vi "Check ref frame has been selected.vi"(6 "Case name string":string, 8 "error in (no error)":errorcluster) -> (0 "error out":errorcluster, 3 "Proceed / Reference frame has been selected":bool)   [LabVIEW 2017]
uses:
  Typedefs/Top level VI states.ctl
  Global Variables/General Globals.vi
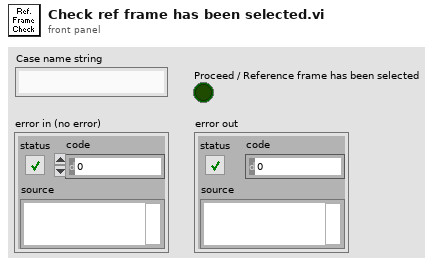
[diagram p1: front panel]
types:
  T1 = typedef "Top level VI states.ctl" = enum16{"None", "Initialise UI", "<STACK PROTOCOL STATES>", "AOL Zstack-START", "AOL Zstack-STOP", "Motor Zstack-START", "Motor Zstack-STOP", "Parameter Sweep-START", "Parameter Sweep-STOP", "<ACQUISITION PROTOCOL STATES> ", "Functional Acquisition-START", "Functional Acquisition-STOP", "Single Plane Acquisition-START", "Single Plane Acquisition-STOP", "Volume Acquisition-START", "Volume Acquisition-STOP", "<LIVE IMAGING PROTOCOL STATES>", "Live Imaging-START", "Live Imaging-STOP", "Live Plane Imaging-START", "Live Plane Imaging-STOP", "Live Volume Imaging-START", "Live Volume Imaging-STOP", "<MOVEMENT CORRECTION PROTOCOL STATES>", "EXIT"}
  T2 = typedef "Reference_Globals.ctl" = cluster{"Refrence data path":path, "Reference Rectangle":i16[][], "AOL Z":dbl, "No of pixels in a miniscan ":i32[], "Threshold":i16[], "No of miniscans":i32[], "Full Frame Size":u16, "Reference Image":T3, "dwelltime":dbl, "Zoom":dbl, "Field of View":dbl, "Z Step":i8, "Z pixels":i32, "Z Lines":u8, "Z Ignore":u8, "Laser":u8}
  T3 = typedef "IMAQ Image.ctl" = refnum<image>
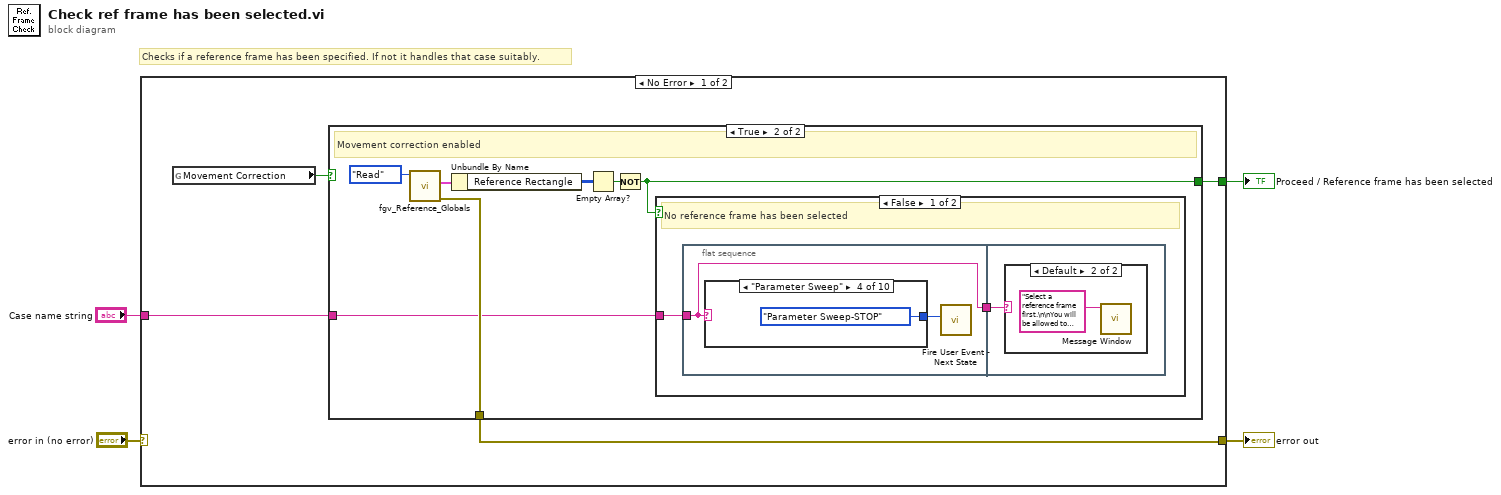
[diagram p0: block diagram]
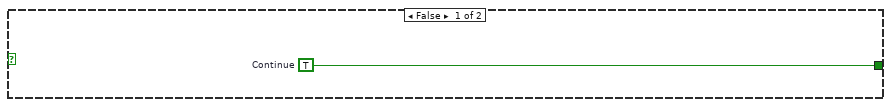
[diagram p2: hidden frame]
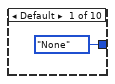
[diagram p3: hidden frame]
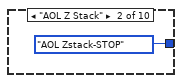
[diagram p4: hidden frame]
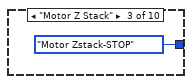
[diagram p5: hidden frame]
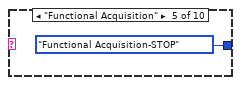
[diagram p6: hidden frame]
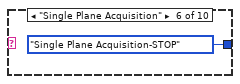
[diagram p7: hidden frame]
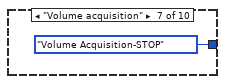
[diagram p8: hidden frame]
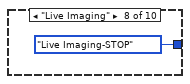
[diagram p9: hidden frame]
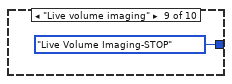
[diagram p10: hidden frame]
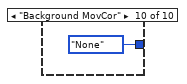
[diagram p11: hidden frame]
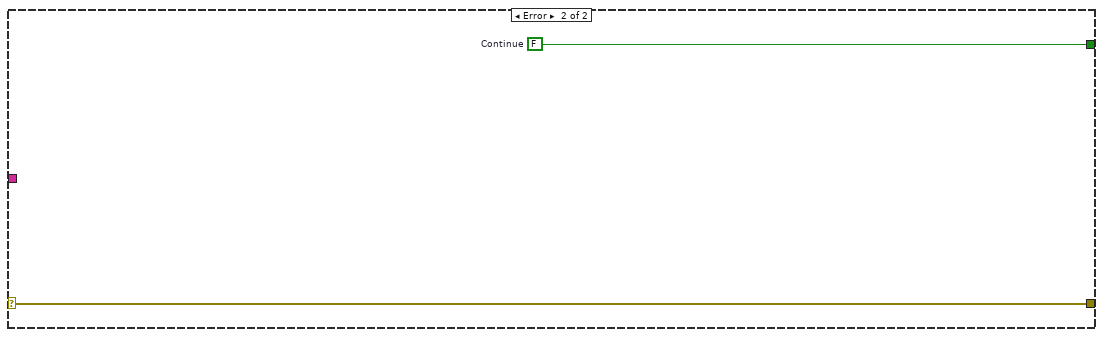
[diagram p14: hidden frame]
diagram:
  # "Checks if a reference frame has been specified. If not it handles that case suitably."
  n1 = case shown="No Error" "error in (no error)" {
    selector: "error in (no error)" -> [_ w34]
    tunnel: [w8 w33] -> w4
    tunnel: [w6 w34] -> w1
    tunnel: "Case name string" -> [w5 _]
    frame No Error {
      n2 = global read "General Globals.vi" "Movement Correction"() -> (w7:bool)
      n3 = case shown="True" w7 {
        tunnel: [w9 w11] -> w8
        tunnel: [_ w12] -> w6
        tunnel: w5 -> [_ w10]
        frame False {
          w9 = TRUE  # Continue
        }
        frame True {
          # "Movement correction enabled"
          n4 = call "fgv_Reference_Globals.vi"("Function"=enum16{"Intialize", "Write", "Read", "Clear"}."Read") -> ("error out"=w12:errorcluster, "Reference Data"=w15:T2)  [unwired: 9 in]
          n5 = Unbundle By Name(w15) -> ("Reference Rectangle"=w14:i16[][])
          n6 = Empty Array?(array=w14) -> (empty?=w13:bool)
          n7 = Not(x=w13) -> (.not. x?=w11:bool)
          n8 = case shown="False" w11 {
            tunnel: w10 -> [w18 _]
            frame False {
              # "No reference frame has been selected"
              n9 = flat-sequence {
                tunnel: w18 -> [w19]
                tunnel: [w19] -> w17
                tunnel: w17 -> [w31]
                frame #0 {
                  n10 = case shown="\"Parameter Sweep\"" w19 {
                    tunnel: [Top_level_VI_states."None" ("event data / imaging mode") Top_level_VI_states."AOL Zstack-STOP" ("event data / imaging mode") Top_level_VI_states."Motor Zstack-STOP" ("event data / imaging mode") Top_level_VI_states."Parameter Sweep-STOP" ("event data / imaging mode") Top_level_VI_states."Functional Acquisition-STOP" ("event data / imaging mode") Top_level_VI_states."Single Plane Acquisition-STOP" ("event data / imaging mode") Top_level_VI_states."Volume Acquisition-STOP" ("event data / imaging mode") Top_level_VI_states."Live Imaging-STOP" ("event data / imaging mode") Top_level_VI_states."Live Volume Imaging-STOP" ("event data / imaging mode") Top_level_VI_states."None" ("event data / imaging mode")] -> w20
                    frame Default {
                    }
                    frame "AOL Z Stack" {
                    }
                    frame "Motor Z Stack" {
                    }
                    frame "Parameter Sweep" {
                    }
                    frame "Functional Acquisition" {
                    }
                    frame "Single Plane Acquisition" {
                    }
                    frame "Volume acquisition" {
                    }
                    frame "Live Imaging" {
                    }
                    frame "Live volume imaging" {
                    }
                    frame "Background MovCor" {
                    }
                  }
                  n11 = call "Fire User Event - Next State.vi"("\"UI Handler loop\" case to execute"=w20) -> ()  [unwired: 10 in, 1 out]
                }
                frame #1 {
                  n12 = case shown="Default" w31 {
                    frame "Background MovCor" {
                    }
                    frame Default {
                      n13 = call "Message Window.vi"("Message string"="Select a reference frame first.\n\nYou will be allowed to select a reference after running the Live Imaging or AOL Z-stack protocol") -> ()  [unwired: 10 in, 1 out]
                    }
                  }
                }
              }
            }
            frame True {
              # "Reference frame has been selected"
            }
          }
        }
      }
    }
    frame Error {
      w33 = FALSE  # Continue
    }
  }
  "Proceed / Reference frame has been selected" <- w4
  "error out" <- w1
